vi "Load.vi"(8 "error in":errorcluster, 10 "Source":string, 11 "ConfiguratorJSON in":refnum<class "Config from JSON.lvclass">) -> (0 "error out":errorcluster, 3 "ConfiguratorJSON out":refnum<class "Config from JSON.lvclass">)   [LabVIEW 2024, in "Config from JSON.lvclass"]
uses:
  Config from JSON.lvclass
  Config from JSON.lvclass/Config from JSON.ctl
  <vilib>/JDP Science/JSONtext/Config Files/Config File.lvclass
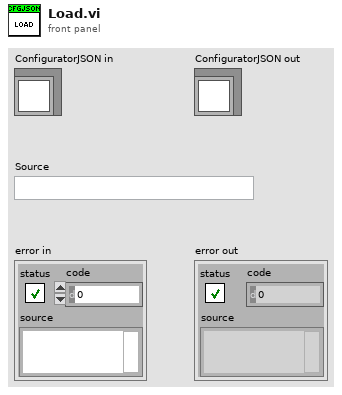
[diagram p1: front panel]
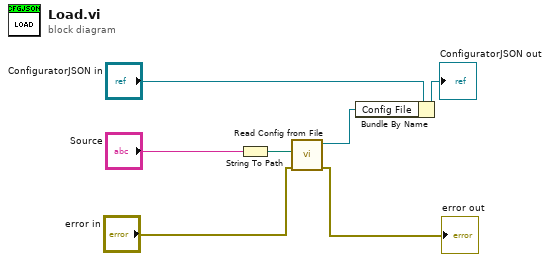
[diagram p0: block diagram]
diagram:
  n1 = String To Path(string="Source") -> (path=w1:path)
  n2 = call <vilib>:"Read Config from File.vi"("error in (no error)"="error in", "config file path"=w1) -> ("error out"=→"error out":errorcluster, "Config File"=w2:refnum<class "Config File.lvclass">)  [unwired: 6 in, 2 out]
  n3 = Bundle By Name(cluster="ConfiguratorJSON in", "Config File"=w2) -> (→"ConfiguratorJSON out":refnum<class "Config from JSON.lvclass">)
